vi "getXYPos.vi"(8 "error in":T1) -> (0 "error out":T1, 2 "y":dbl format="%#_g µm", 3 "x":dbl format="%#_g µm")   [LabVIEW 2016]
doc: "returns the current X- and Y-coordinates of the scanner in µm."
uses:
  Controls/Error_Out.ctl
  Files_ASC500/DLL/ASC500_RemoteControlV27.dll
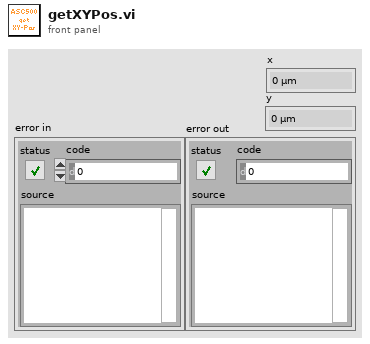
[diagram p1: front panel]
types:
  T1 = typedef "Error_Out.ctl" = errorcluster
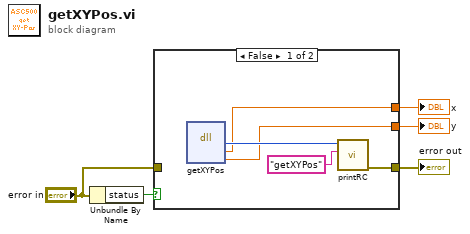
[diagram p0: block diagram]
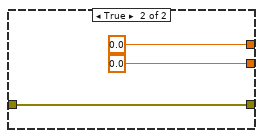
[diagram p2: hidden frame]
diagram:
  n1 = Unbundle By Name("error in") -> ("status"=w5:bool)
  n2 = case shown="False" w5 {
    tunnel: "error in" -> [_ w11]
    tunnel: [w9 0.0] -> w3
    tunnel: [w8 0.0] -> w2
    tunnel: [w6 w11] -> w1
    frame False {
      n3 = dll-call lib="G:/SCMOperations/Share/ELE/Produkt Information/ASC500/04 Remote Control/02 development versions/2018Nov06/Files_ASC500/DLL/ASC500_RemoteControlV27.dll" fn="getXYPos"() -> ("RC"=w10:i32, "x"=w9:dbl, "y"=w8:dbl)  [unwired: 5 in, 2 out]
      n4 = call "printRC.vi"("additional information"="getXYPos", "RC"=w10) -> ("error out"=w6:T1)  [unwired: 9 in]
    }
    frame True {
    }
  }
  "x" <- w3
  "y" <- w2
  "error out" <- w1
